vi "Autonomous.vi"   [LabVIEW 2018]
doc: "This VI starts when autonomous period begins, and will automatically be terminated when it ends. You can carry out timed or sensor driven operations directly to I/O or to subsystems without needing to return to the caller."
uses:
  <vilib>/Rock Robotics/WPI/Solenoid/WPI_SolenoidValue.ctl
  <vilib>/Rock Robotics/WPI/Utilities/WPI_GetSetVariantRefNum.vi
  <vilib>/Rock Robotics/Network Tables/NT Read String.vi
  Framework/Robot Global Data.vi
types:
  T1 = typedef "WPI_SolenoidValue.ctl" = enum16{"Off", "On", "Forward", "Reverse"}
  T2 = typedef "WPI_JoystickDevRef.ctl" = cluster{"Device":T3}
  T3 = typedef "WPI_JoystickDeviceEnum.ctl" = enum16{"USB 0", "USB 1", "USB 2", "USB 3", "USB 4", "USB 5"}
  T4 = typedef "Command Status Info.ctl" = cluster{"Name":string, "Status":T5, "notifier out":T6}
  T5 = typedef "Completion Status.ctl" = enum16{"Successful", "Aborted", "Incomplete"}
  T6 = typedef "Completion Notifier.ctl" = refnum<notifier>
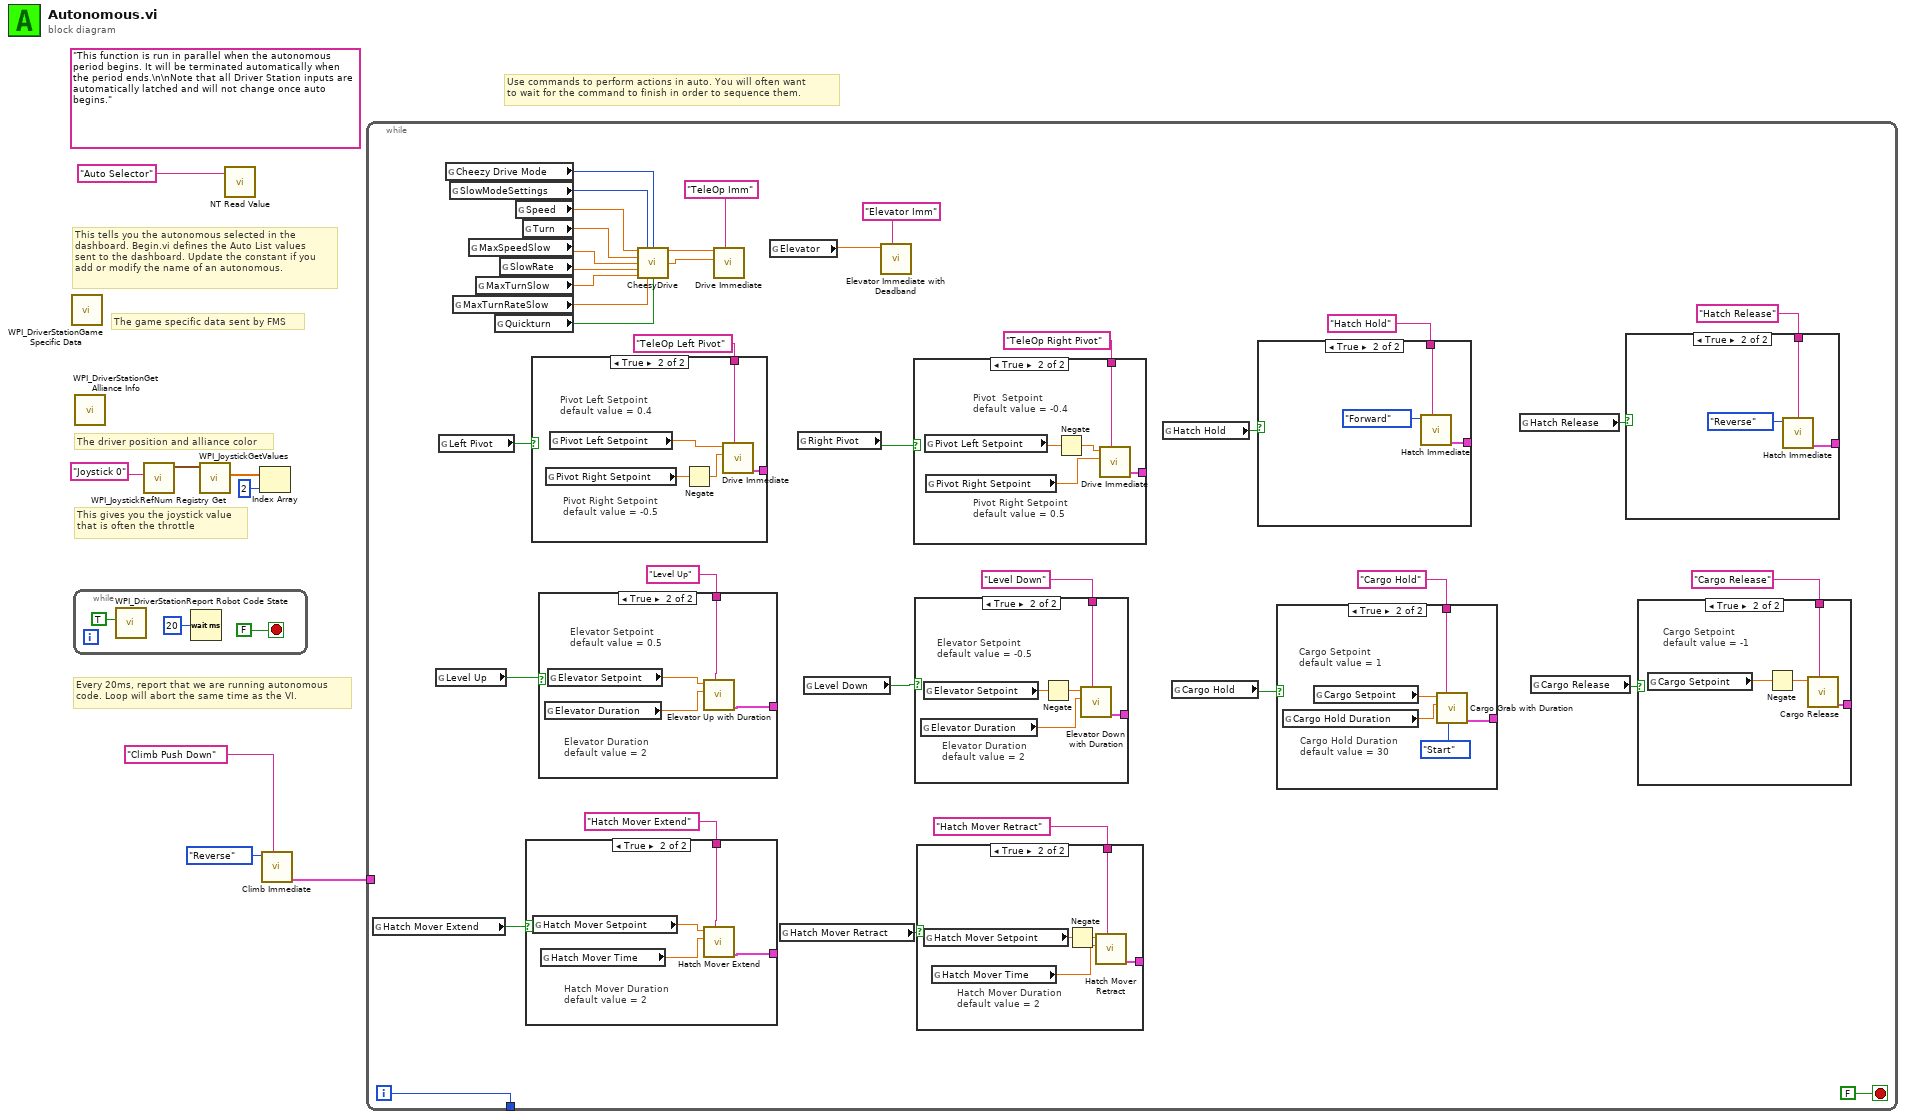
[diagram p0: block diagram]
diagram:
  (unwired) "This function is run in parallel when the autonomous period begins. It will be terminated automatically when the period ends.\n\nNote that all Driver Station inputs are automatically latched and will not change once auto begins."
  # "The game specific data sent by FMS"
  # "This tells you the autonomous selected in the \ndashboard. Begin.vi defines the Auto List values\nsent to the dashboard. Update the constant if you\nadd or modify the name of an autonomous."
  # "Every 20ms, report that we are running autonomous\ncode. Loop will abort the same time as the VI."
  # "This gives you the joystick value\nthat is often the throttle"
  # "Use commands to perform actions in auto. You will often want\nto wait for the command to finish in order to sequence them."
  # "The driver position and alliance color"
  n1 = call <vilib>:"WPI_DriverStationGame Specific Data.vi"() -> ()  [unwired: 11 in, 1 out]
  n2 = while {
    stop <- FALSE stop-if-true
    n3 = call <vilib>:"WPI_DriverStationReport Robot Code State.vi"("Autonomous"=TRUE) -> ()  [unwired: 10 in, 1 out]
    n4 = Wait (ms)(milliseconds to wait=u32 20) -> ()  [unwired: 1 out]
  }
  n5 = call <vilib>:"WPI_DriverStationGet Alliance Info.vi"() -> ()  [unwired: 12 out]
  n6 = call <vilib>:"WPI_JoystickRefNum Registry Get.vi"("refnum name"="Joystick 0") -> ("JoystickDevRef"=w7:T2)  [unwired: 1 in, 9 out]
  n7 = call <vilib>:"WPI_JoystickGetValues.vi"("JoystickDevRef"=w7) -> ("Axes"=w6:dbl[])  [unwired: 6 in, 4 out]
  n8 = call-poly <vilib>:"NT Read Value.vi"("Name"="Auto Selector") -> ()  [unwired: 9 in, 2 out]
  n9 = Index Array(array=w6, index=2) -> ()  [unwired: 1 out]
  n10 = call "Climb Immediate.vi"("Description"="Climb Push Down", "Climb Action"=WPI_SolenoidValue."Reverse") -> ("Command Info Out"=w2:T4)  [unwired: 9 in]
  n11 = while {
    tunnel: [w12] -> _
    tunnel: w2 -> [_]
    i -> [w12]
    stop <- FALSE stop-if-true
    n12 = global read "Robot Global Data.vi" "Hatch Mover Extend"() -> (w19:bool)
    n13 = global read "Robot Global Data.vi" "Level Up"() -> (w24:bool)
    n14 = global read "Robot Global Data.vi" "Left Pivot"() -> (w30:bool)
    n15 = global read "Robot Global Data.vi" "Cheezy Drive Mode"() -> (w44:u32)
    n16 = global read "Robot Global Data.vi" "SlowModeSettings"() -> (w34:i32)
    n17 = global read "Robot Global Data.vi" "MaxTurnRateSlow"() -> (w36:dbl)
    n18 = global read "Robot Global Data.vi" "MaxSpeedSlow"() -> (w39:dbl)
    n19 = global read "Robot Global Data.vi" "MaxTurnSlow"() -> (w37:dbl)
    n20 = global read "Robot Global Data.vi" "Quickturn"() -> (w35:bool)
    n21 = global read "Robot Global Data.vi" "SlowRate"() -> (w38:dbl)
    n22 = global read "Robot Global Data.vi" "Speed"() -> (w41:dbl)
    n23 = global read "Robot Global Data.vi" "Turn"() -> (w40:dbl)
    n24 = case shown="True" w19 {
      tunnel: [_ w65] -> _
      tunnel: "Hatch Mover Extend" ("Description") -> [_ w64]
      frame False {
      }
      frame True {
        # "Hatch Mover Duration\ndefault value = 2"
        n25 = global read "Robot Global Data.vi" "Hatch Mover Setpoint"() -> (w63:dbl)
        n26 = global read "Robot Global Data.vi" "Hatch Mover Time"() -> (w62:dbl)
        n27 = call "Hatch Mover Extend.vi"("Description"=w64, "Duration (s)"=w62, "Setpoint"=w63) -> ("Command Info Out"=w65:T4)  [unwired: 8 in]
      }
    }
    n28 = case shown="True" w30 {
      tunnel: [_ w90] -> _
      tunnel: "TeleOp Left Pivot" ("Description") -> [_ w89]
      frame False {
      }
      frame True {
        # "Pivot Right Setpoint\ndefault value = -0.5"
        # "Pivot Left Setpoint\ndefault value = 0.4"
        n29 = global read "Robot Global Data.vi" "Pivot Right Setpoint"() -> (w87:dbl)
        n30 = global read "Robot Global Data.vi" "Pivot Left Setpoint"() -> (w88:dbl)
        n31 = Negate(x=w87) -> (-x=w86:dbl)
        n32 = call "Drive Immediate.vi"("Description"=w89, "Right Setpoint"=w86, "Left Setpoint"=w88) -> ("Command Info Out"=w90:T4)  [unwired: 8 in]
      }
    }
    n33 = case shown="True" w24 {
      tunnel: [_ w74] -> _
      tunnel: "Level Up" ("Description") -> [_ w73]
      frame False {
      }
      frame True {
        # "Elevator Setpoint\ndefault value = 0.5"
        # "Elevator Duration\ndefault value = 2"
        n34 = global read "Robot Global Data.vi" "Elevator Duration"() -> (w71:dbl)
        n35 = global read "Robot Global Data.vi" "Elevator Setpoint"() -> (w72:dbl)
        n36 = call "Elevator Up with Duration.vi"("Description"=w73, "Duration (s)"=w71, "Setpoint"=w72) -> ("Command Info Out"=w74:T4)  [unwired: 8 in]
      }
    }
    n37 = call "CheesyDrive.vi"("Throttle"=w41, "SlowModeSettings"=w34, "SlowMode"=w44, "Wheel"=w40, "MaxSpeedSlow"=w39, "SlowRate"=w38, "MaxTurnSlow"=w37, "MaxTurnRateSlow"=w36, "Quickturn"=w35) -> ("Left PWM"=w43:dbl, "Right PWM"=w42:dbl)  [unwired: 5 in]
    n38 = call "Drive Immediate.vi"("Description"="TeleOp Imm", "Right Setpoint"=w42, "Left Setpoint"=w43) -> ()  [unwired: 8 in, 1 out]
    n39 = global read "Robot Global Data.vi" "Elevator"() -> (w46:dbl)
    n40 = global read "Robot Global Data.vi" "Hatch Mover Retract"() -> (w20:bool)
    n41 = global read "Robot Global Data.vi" "Right Pivot"() -> (w31:bool)
    n42 = global read "Robot Global Data.vi" "Level Down"() -> (w23:bool)
    n43 = call "Elevator Immediate with Deadband.vi"("Description"="Elevator Imm", "Setpoint"=w46) -> ()  [unwired: 9 in, 1 out]
    n44 = case shown="True" w31 {
      tunnel: [_ w85] -> _
      tunnel: "TeleOp Right Pivot" ("Description") -> [_ w84]
      frame False {
      }
      frame True {
        # "Pivot Right Setpoint\ndefault value = 0.5"
        # "Pivot  Setpoint\ndefault value = -0.4"
        n45 = global read "Robot Global Data.vi" "Pivot Left Setpoint"() -> (w82:dbl)
        n46 = global read "Robot Global Data.vi" "Pivot Right Setpoint"() -> (w83:dbl)
        n47 = Negate(x=w82) -> (-x=w81:dbl)
        n48 = call "Drive Immediate.vi"("Description"=w84, "Right Setpoint"=w83, "Left Setpoint"=w81) -> ("Command Info Out"=w85:T4)  [unwired: 8 in]
      }
    }
    n49 = case shown="True" w23 {
      tunnel: "Level Down" ("Description") -> [_ w70]
      tunnel: [_ w69] -> _
      frame False {
      }
      frame True {
        # "Elevator Duration\ndefault value = 2"
        # "Elevator Setpoint\ndefault value = -0.5"
        n50 = global read "Robot Global Data.vi" "Elevator Duration"() -> (w67:dbl)
        n51 = global read "Robot Global Data.vi" "Elevator Setpoint"() -> (w68:dbl)
        n52 = Negate(x=w68) -> (-x=w66:dbl)
        n53 = call "Elevator Down with Duration.vi"("Description"=w70, "Duration (s)"=w67, "Setpoint"=w66) -> ("Command Info Out"=w69:T4)  [unwired: 8 in]
      }
    }
    n54 = case shown="True" w20 {
      tunnel: "Hatch Mover Retract" ("Description") -> [_ w61]
      tunnel: [_ w60] -> _
      frame False {
      }
      frame True {
        # "Hatch Mover Duration\ndefault value = 2"
        n55 = global read "Robot Global Data.vi" "Hatch Mover Setpoint"() -> (w59:dbl)
        n56 = global read "Robot Global Data.vi" "Hatch Mover Time"() -> (w58:dbl)
        n57 = Negate(x=w59) -> (-x=w57:dbl)
        n58 = call "Hatch Mover Retract.vi"("Description"=w61, "Duration (s)"=w58, "Setpoint"=w57) -> ("Command Info Out"=w60:T4)  [unwired: 8 in]
      }
    }
    n59 = global read "Robot Global Data.vi" "Hatch Hold"() -> (w26:bool)
    n60 = global read "Robot Global Data.vi" "Cargo Hold"() -> (w15:bool)
    n61 = case shown="True" w26 {
      tunnel: "Hatch Hold" ("Description") -> [_ w80]
      tunnel: [_ w79] -> _
      frame False {
      }
      frame True {
        n62 = call "Hatch Immediate.vi"("Description"=w80, "Hatch Action"=WPI_SolenoidValue."Forward") -> ("Command Info Out"=w79:T4)  [unwired: 9 in]
      }
    }
    n63 = case shown="True" w15 {
      tunnel: [_ w56] -> _
      tunnel: "Cargo Hold" ("Description") -> [_ w55]
      frame False {
      }
      frame True {
        # "Cargo Hold Duration\ndefault value = 30"
        # "Cargo Setpoint\ndefault value = 1"
        n64 = global read "Robot Global Data.vi" "Cargo Hold Duration"() -> (w52:dbl)
        n65 = global read "Robot Global Data.vi" "Cargo Setpoint"() -> (w54:dbl)
        n66 = call "Cargo Grab with Duration.vi"("Synchronization"=enum16{"Start", "Wait"}."Start", "Description"=w55, "Duration (s)"=w52, "Setpoint"=w54) -> ("Command Info Out"=w56:T4)  [unwired: 7 in]
      }
    }
    n67 = global read "Robot Global Data.vi" "Hatch Release"() -> (w27:bool)
    n68 = global read "Robot Global Data.vi" "Cargo Release"() -> (w14:bool)
    n69 = case shown="True" w27 {
      tunnel: "Hatch Release" ("Description") -> [_ w77]
      tunnel: [_ w76] -> _
      frame False {
      }
      frame True {
        n70 = call "Hatch Immediate.vi"("Description"=w77, "Hatch Action"=WPI_SolenoidValue."Reverse") -> ("Command Info Out"=w76:T4)  [unwired: 9 in]
      }
    }
    n71 = case shown="True" w14 {
      tunnel: [_ w51] -> _
      tunnel: "Cargo Release" ("Description") -> [_ w50]
      frame False {
      }
      frame True {
        # "Cargo Setpoint\ndefault value = -1"
        n72 = global read "Robot Global Data.vi" "Cargo Setpoint"() -> (w49:dbl)
        n73 = Negate(x=w49) -> (-x=w48:dbl)
        n74 = call "Cargo Release.vi"("Description"=w50, "Setpoint"=w48) -> ("Command Info Out"=w51:T4)  [unwired: 9 in]
      }
    }
  }
